vi "Display Synchronous.vi"(6 "Sampling":T1={"Fs"=204789.0, "#s"=15753} {"Fs" format="%#_13g"}, 8 "error in (no error)":errorcluster, 9 "phase (°)":dbl, 10 "frequency (Hz)":dbl, 11 "Input Waveforms":waveform(dbl)[](array[waveform])) -> (0 "error out":errorcluster, 3 "Output Waveforms":waveform(dbl)[](array[waveform]))   [LabVIEW 2019, in "Instrument.Lockin.lvlib" / "Instrument UI.Lockin.lvclass"]
uses:
  Instrument UI.Lockin.lvclass
  Instrument.DAQ/Typedefs/DAQ.Sampling.Sampling--Cluster.ctl
  <vilib>/PRIrvin/XY Utilities/subVIs/Circular Buffer (waveforms).vi
  <vilib>/PRIrvin/XY Utilities/xy_utilities.lvlib
  Instrument.DAQ/Instrument.DAQ.lvclass
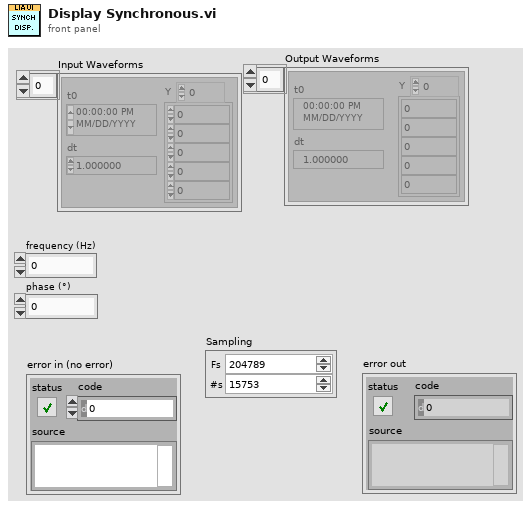
[diagram p1: front panel]
types:
  T1 = typedef "Instrument.Lockin.lvlib/Instrument.DAQ.lvclass/DAQ.Sampling.Sampling--Cluster.ctl" = cluster{"Fs":dbl, "#s":i32}
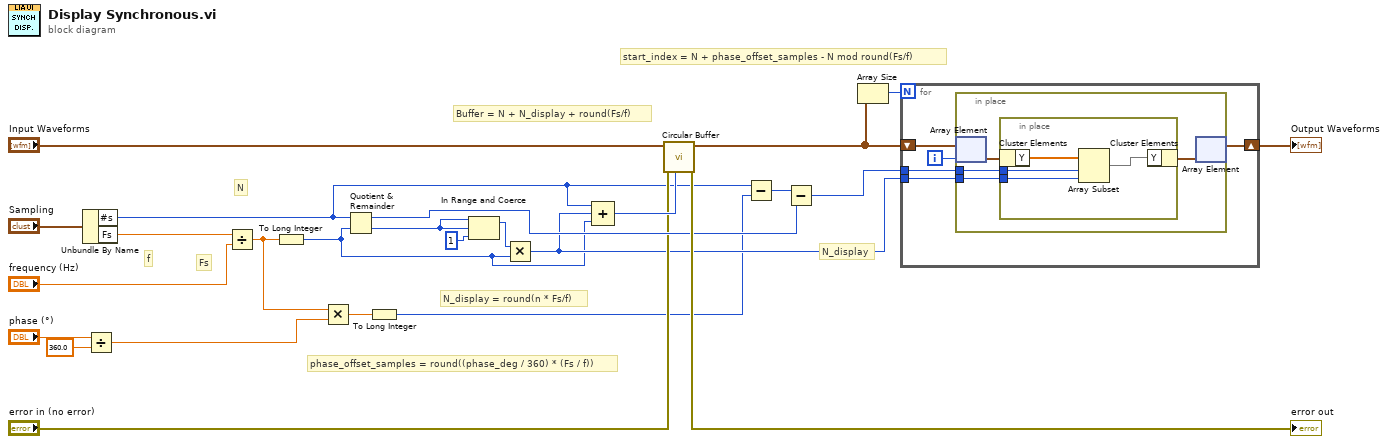
[diagram p0: block diagram]
diagram:
  # "N_display"
  # "Buffer = N + N_display + round(Fs/f)"
  # "N_display = round(n * Fs/f)"
  # "start_index = N + phase_offset_samples - N mod round(Fs/f)"
  # "phase_offset_samples = round((phase_deg / 360) * (Fs / f))"
  # "N"
  # "Fs"
  # "f"
  n1 = Unbundle By Name("Sampling") -> ("#s"=w3:i32, "Fs"=w14:dbl)
  n2 = Divide(x="phase (°)", y=360.0) -> (x/y=w12:dbl)
  n3 = Divide(x=w14, y="frequency (Hz)") -> (x/y=w7:dbl)
  n4 = To Long Integer(number=w7) -> (32bit integer=w1:i32)
  n5 = Multiply(x=w7, y=w12) -> (x*y=w11:dbl)
  n6 = Quotient & Remainder(x=w3, y=w1) -> (x-y*floor(x/y)=w9:i32, floor(x/y)=w23:i32)
  n7 = To Long Integer(number=w11) -> (32bit integer=w2:i32)
  n8 = In Range and Coerce(upper limit=w23, x=w23, lower limit=1) -> (coerced(x)=w22:i32)  [unwired: 1 out]
  n9 = Multiply(x=w22, y=w1) -> (x*y=w4:i32)
  n10 = Compound Arithmetic op=ADD(w3, w4, w1) -> (w17:i32)
  n11 = call-poly <vilib>:"Circular Buffer.vi"("History Length [1024]"=w17, "error in"="error in (no error)", "Waveform in"="Input Waveforms") -> ("error out"=→"error out":errorcluster, "Waveform out"=w18:waveform(dbl)[])  [unwired: 7 in]
  n12 = Subtract(x=w3, y=w2) -> (x-y=w6:i32)
  n13 = Subtract(x=w6, y=w9) -> (x-y=w5:i32)
  n14 = Array Size(array=w18) -> (size(s)=w20:i32)
  n15 = for {
    N: w20 -> [_]
    shift-right: [w28] -> w19
    shift-left: w18 -> [w29]
    tunnel: w5 -> [w27]
    tunnel: w4 -> [w26]
    i -> [w30]
    n16 = in-place {
      in-place-border: w27 -> [w32]
      in-place-border: w26 -> [w31]
      n17 = in-place-array #1(w29, w30) -> (w34:waveform(dbl))
      n18 = in-place {
        in-place-border: w32 -> [w36]
        in-place-border: w31 -> [w35]
        n19 = in-place-cluster #2(w34) -> ("Y"=w38:dbl[])
        n20 = Array Subset(array=w38, index=w36, length=w35) -> (w37:dbl[])
        n21 = in-place-cluster #2("Y"=w37) -> (w33:waveform(dbl))
      }
      n22 = in-place-array #1(w33) -> (w28:waveform(dbl)[])  [unwired: 1 out]
    }
  }
  "Output Waveforms" <- w19
